vi "Keithley 6430 Sweep.vi"() -> ()   [LabVIEW 2019]
panel:
  in  "stop":bool
  in  "Log Sweep?":bool
  in  "Compliance Voltage":dbl=10.0 format="%.3f"
  in  "Sweep Time (H:M:S)":dbl format="%<%H:%M:%S>t"
  in  "Stop Current":dbl=0.007 min=-0.007 max=0.007 format="%^.3e"
  in  "Start Current":dbl min=-0.105 max=0.007 format="%^.3e"
  in  "Output Off":bool
  in  "Start Sweep":bool
  in  "Setup":bool
  in  "VISA resource name":refnum<visa-resource-name>
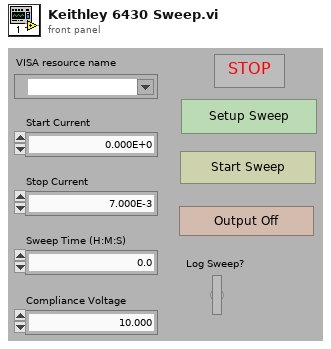
[diagram p1: front panel]
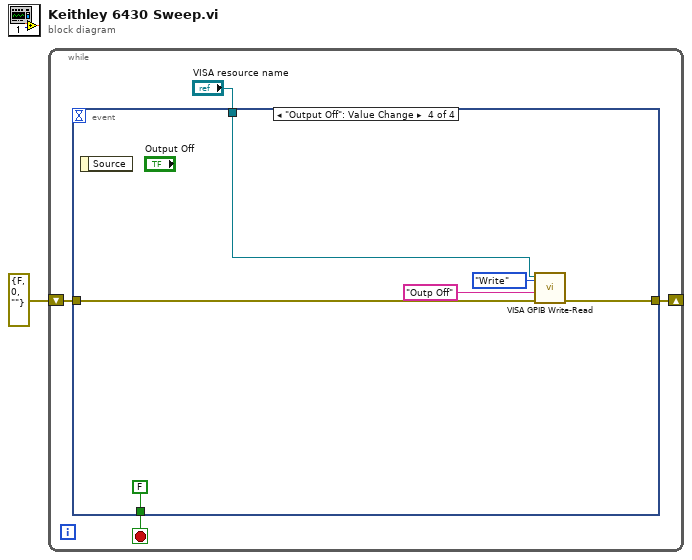
[diagram p0: block diagram]
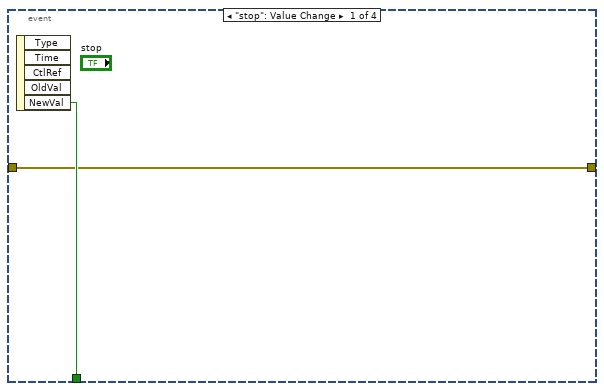
[diagram p2: hidden frame]
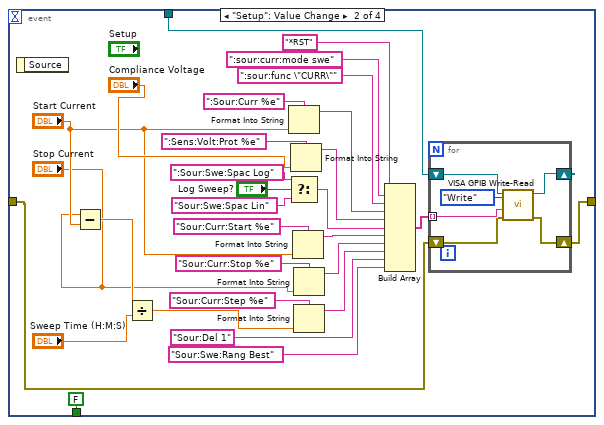
[diagram p3: hidden frame]
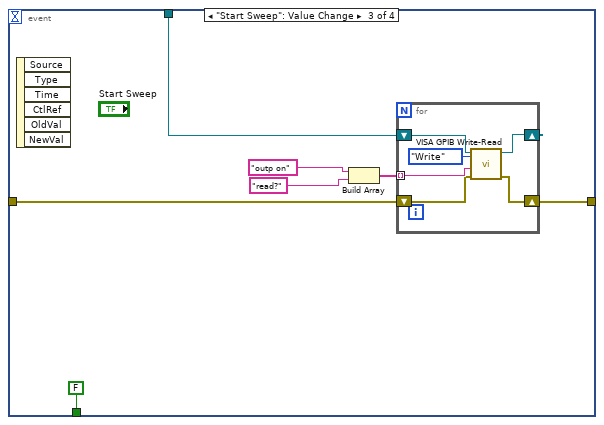
[diagram p4: hidden frame]
diagram:
  n1 = while {
    shift-right: [w3] -> _
    shift-left: errorcluster {"status"=FALSE, "code"=0, "source"=""} ("error out") -> [w2]
    stop <- w4 stop-if-true
    n2 = event shown="[3] \"Output Off\": Value Change" {
      selector: _ -> [_ _ _ _]
      dyn-events: _ -> [_ _ _ _]
      timeout: _ -> [_ _ _ _]
      tunnel: "VISA resource name" -> [_ w21 w50 w62]
      tunnel: [w7 FALSE ("NewVal") FALSE ("NewVal") FALSE ("NewVal")] -> w4
      tunnel: [w6 w16 w44 w58] -> w3
      tunnel: w2 -> [w6 w15 w45 w57]
      event "stop": Value Change {
        n3 = event-data() -> ("NewVal"=w7:bool)  [unwired: 1 in, 4 out]
      }
      event "Setup": Value Change {
        n4 = event-data() -> ()  [unwired: 1 in, 1 out]
        n5 = Subtract(x="Stop Current", y="Start Current") -> (x-y=w14:dbl)
        n6 = Divide(x=w14, y="Sweep Time (H:M:S)") -> (x/y=w18:dbl)
        n7 = Format Into String(format string=":Sour:Curr %e", "Start Current") -> (resulting string=w30:string)  [unwired: 2 in, 1 out]
        n8 = Select(t=":Sour:Swe:Spac Log", s="Log Sweep?", f="Sour:Swe:Spac Lin") -> (s? t:f=w28:string)
        n9 = Format Into String(format string=":Sens:Volt:Prot %e", "Compliance Voltage") -> (resulting string=w29:string)  [unwired: 2 in, 1 out]
        n10 = Format Into String(format string="Sour:Curr:Start %e", "Start Current") -> (resulting string=w27:string)  [unwired: 2 in, 1 out]
        n11 = Format Into String(format string="Sour:Curr:Stop %e", "Stop Current") -> (resulting string=w26:string)  [unwired: 2 in, 1 out]
        n12 = Format Into String(format string="Sour:Curr:Step %e", w18) -> (resulting string=w25:string)  [unwired: 2 in, 1 out]
        n13 = Build Array("*RST", ":sour:curr:mode swe" ("element"), ":sour:func \"CURR\"" ("element"), w30, w29, w28, w27, w26, w25, "Sour:Del 1", "Sour:Swe:Rang Best") -> (w22:string[])
        n14 = for {
          tunnel: w22 -> [w42] mode=indexing
          shift-right: [w40] -> _
          shift-left: w21 -> [w41]
          shift-right: [w38] -> w16
          shift-left: w15 -> [w39]
          n15 = call "VISA GPIB Write-Read.vi"("error in (no error)"=w39, "Command"=w42, "Action"=enum16{"Write", "Read", "Write & Read"}."Write", "VISA resource name"=w41) -> ("error out"=w38:errorcluster, "dup VISA Session"=w40:refnum<visa-resource-name>)  [unwired: 4 in, 2 out]
        }
      }
      event "Start Sweep": Value Change {
        n16 = event-data() -> ()  [unwired: 1 in, 6 out]
        n17 = Build Array("outp on", "read?") -> (w49:string[])
        n18 = for {
          tunnel: w49 -> [w55] mode=indexing
          shift-right: [w53] -> _
          shift-left: w50 -> [w54]
          shift-right: [w51] -> w44
          shift-left: w45 -> [w52]
          n19 = call "VISA GPIB Write-Read.vi"("error in (no error)"=w52, "Command"=w55, "Action"=enum16{"Write", "Read", "Write & Read"}."Write", "VISA resource name"=w54) -> ("error out"=w51:errorcluster, "dup VISA Session"=w53:refnum<visa-resource-name>)  [unwired: 4 in, 2 out]
        }
      }
      event "Output Off": Value Change {
        n20 = event-data() -> ()  [unwired: 1 in, 1 out]
        n21 = call "VISA GPIB Write-Read.vi"("error in (no error)"=w57, "Command"="Outp Off", "Action"=enum16{"Write", "Read", "Write & Read"}."Write", "VISA resource name"=w62) -> ("error out"=w58:errorcluster)  [unwired: 4 in, 3 out]
      }
    }
  }
